vi "BLM Command.vi"(5 "Timeout Limit":sgl=0.1 format="%.2f", 6 "Motor Address":string="0", 7 "error in (no error)":errorcluster, 8 "Read Echo?":bool, 9 "Command":string="RE", 10 "Port Address":refnum<visa-resource-name>) -> (0 "error out":errorcluster, 1 "Response":string, 2 "Timeout":bool, 3 "Port Address Out":refnum<visa-resource-name>, 4 "Delta Time":u32)   [LabVIEW 2018]
uses:
  IMS Stepper Controller/Serial Support VISA.llb/Serial Actions.ctl
panel:
  # "Send command RE (reset) to identify\nASRL address: proper responce is %"
  # "will give error 5202\non MN command (BLM)"
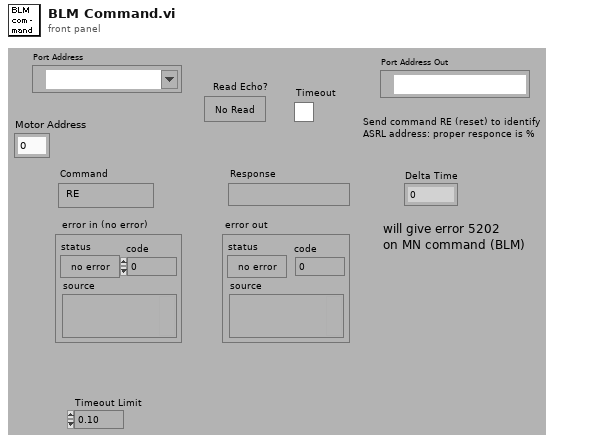
[diagram p1: front panel]
types:
  T1 = typedef "Serial Actions.ctl" = enum16{"Init", "Break", "Clear Buffer", "Write", "Read", "N Bytes", "Lock", "Unlock", "Close"}
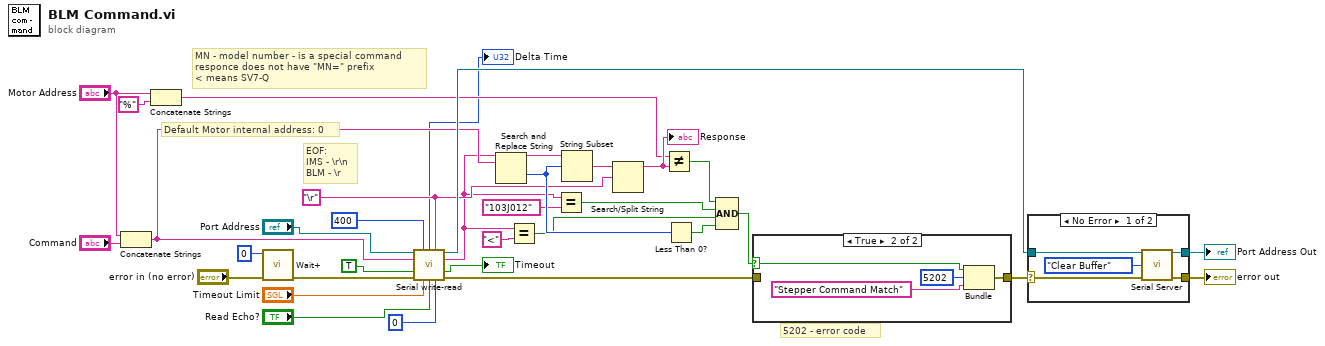
[diagram p0: block diagram]
diagram:
  w23 = "\r" ("EOT Chars (cr/lf)")
  # "Default Motor internal address: 0"
  # "MN - model number - is a special command\nresponce does not have \"MN=\" prefix\n< means SV7-Q"
  # "EOF:\nIMS - \\r\\n\nBLM - \\r"
  # "5202 - error code"
  n1 = Concatenate Strings("Motor Address", "Command") -> (w17:string)
  n2 = Concatenate Strings("Motor Address", "%" ("x")) -> (w19:string)
  n3 = call "Wait+.vi"("Error In"="error in (no error)", "milliseconds to wait"=u32 0) -> ("Error Out"=w32:errorcluster)  [unwired: 4 in, 1 out]
  n4 = call "Serial write-read.vi"("VISA Resource Name"="Port Address", "Max Char to Read"=u32 400, "EOT Chars (cr/lf)"=w23, "String To Send"=w17, "Clear Buffer?"=TRUE, "error in (no error)"=w32, "Timeout Limit"="Timeout Limit", "Read Echo?"="Read Echo?", "milliseconds to wait"=u32 0) -> ("mSec"=→"Delta Time":u32, "dup VISA Resource Name"=w29:refnum<visa-resource-name>, "Serial Read"=w10:string, "Timeout"=→"Timeout":bool, "error out"=w31:errorcluster)  [unwired: 1 in, 1 out]
  n5 = Search and Replace String(input string=w10, search string=w17) -> (result string=w25:string, offset past replacement=w24:i32)  [unwired: 6 in, 2 out]
  n6 = Equal?(x=w10, y="<" ("x")) -> (x = y?=w14:bool)
  n7 = Equal?(x=w10, y="103J012" ("x")) -> (x = y?=w11:bool)
  n8 = String Subset(string=w25, offset (0)=w24) -> (substring=w26:string)  [unwired: 1 in]
  n9 = Search/Split String(string=w26, search string/char (-)=w23) -> (substring before match=w21:string)  [unwired: 1 in, 2 out]
  "Response" <- w21
  n10 = Not Equal?(x=w19, y=w21) -> (x != y?=w15:bool)
  n11 = Less Than 0?(x=w24) -> (x < 0?=w27:bool)
  n12 = Compound Arithmetic op=AND(w15, w11, w14, w27) -> (w22:bool)
  n13 = case shown="True" w22 {
    selector: w22 -> [_ w38]
    tunnel: [w35 w39] -> w9
    tunnel: w31 -> [w35 _]
    frame False {
    }
    frame True {
      n14 = Bundle(w38, 5202, "Stepper Command Match") -> (w39:errorcluster)  [unwired: 1 in]
    }
  }
  n15 = case shown="No Error" w9 {
    selector: w9 -> [w41 w46]
    tunnel: w29 -> [w43 w45]
    tunnel: [w42 w46] -> w28
    tunnel: [w40 w45] -> w8
    frame No Error {
      n16 = call "Serial Server.vi"("VISA Resource Name"=w43, "Action"=Serial_Actions."Clear Buffer", "error in (no error)"=w41) -> ("dup VISA Resource Name"=w40:refnum<visa-resource-name>, "error out"=w42:errorcluster)  [unwired: 8 in, 3 out]
    }
    frame Error {
    }
  }
  "error out" <- w28
  "Port Address Out" <- w8
